vi "Fit EPR Spectra (QSM)-Rev2.vi"(8 "Spectral Data In":T6={"PDT Amp [v]"=0.0, "RIS Amp [v]"=0.0, "B-Field"=[], "All In-Phase Scan Spectra"=[], "Model Select"=enum."OneCompRISTwoPDT", "Fit Each Scan"=FALSE, "PDT Center [g]"=0.0, "In-Phase Average Spectra"=[], "In-Phase Median Spectra"=[], "Out-Phase Median Spectra"=[], "Out-Phase Average Spectra"=[], "Fit Spectra"=[], "Fit No-Baseline Spectra"=[], "All Out-Phase Scan Spectra"=[], "Baseline Offset Correction"=FALSE, "In-Phase Offset [v]"=0.0, "Out-Phase Offset [v]"=0.0, "Ch2 Input\n(Balance)"=[], "Ch3 Input\n(Phase)"=[], "Ch4 Input\n(AFC)"=[], "Fit Pars"=[], "Fit Pars Errors"=[], "Fit Pars Labels"=[], "Raw Scan DAQ Data"=[], "Bad Scans Indicies"=[], "Good In-Phase Scan Spectra"=[], "Good Out-Phase Scan Spectra"=[], "Bad In-Phase Scan Spectra"=[], "Bad Out-Phase Scan Spectra"=[], "Number of bad scans"=0, "Fit History"=[], "PDT Amp. History/Set [v]"=[], "RIS Amp. History/Set [v]"=[], "RIS Amp. History/Scan [v]"=[], "All Shifted B-Fields"=[], "Good Shifted B-Fields"=[], "Ch5 Input\n(SpO2)"=[], "Ch6 Input\n(BPM)"=[], "Global SNR"=0.0, "Fit Error History"=[], "SNR History"=[]} {"Global SNR" min=0.0; "PDT Center [g]" min=0.0; "RIS Amp [v]" min=0.0}, 9 "Measurement Information":T1={"Comments"="", "Directory Input"="", "Data file path"=path "C:/Data/EPR Data", "Scripting File"=path "C:/Data/Configuration Script.csv", "Save Data"=FALSE, "Tooth size (d11) [mm]"=0.0, "Tooth size (d12) [mm]"=0.0, "Tooth size (d21) [mm]"=0.0, "Tooth size (d22) [mm]"=0.0, "Dose of Tooth [Gy]"=0.0, "Safe Shutdown?"=FALSE, "Gases Available"=[], "Database Username"="", "Database Password"="", "Database Login URL"="", "Database Upload URL"="", "Database Success URL"="", "Database XML URL"="", "Database Resonator URL"="", "Session Number"=0, "Set #"=0, "Resonator Operator"="", "Session Type"="", "Tooth/Sample ID"="", "Volunteer ID"="", "Computer Operator"="", "Volunteer Type"="", "Site/Tooth Selection (T8,T9)"="", "Resonator"="", "Measurement Site"="", "Non-standard session?"=FALSE, "EPR DAQ Version"="", "Session Path"=path "C:/Data/EPR Data", "Chosen Applied State"="", "Chosen Initial State"="", "Time of Transition"="", "DAQ Mode"=enum."Engineering", "pO2/Scan [mmHg]"=[], "pO2/Set [mmHg]"=[], "Linewidth (HWHM)/Scan [Gauss]"=[], "Linewidth (HWHM)/Set [Gauss]"=[], "pO2 Conversion"="", "Dose Calibration Cluster"={"Dose Response"={"grand_mean"=0.0292016, "slope"=0.0188720543}, "Dose Correction"={"Sex"=1, "a0"=7.719669421, "a1"=-2.746550736, "a2"=-0.186490355, "a3"=0.041922063, "a4"=-0.849147359, "a5"=0.14330063, "a6"=0.019930219, "A_n"=40.0, "H_n"=10.12, "Dose Correction"=FALSE}, "Dose Reporting"={"Reporting is"=TRUE, "sd_threshold [AU]"=0.06, "sd_model [Gy]"=0.66, "dosimetric_threshold [Gy]"=2.0, "Add intrasession errors is"=FALSE, "Prior Radiation?"=FALSE}}, "OxyChip Slope"=0.0, "OxyChip Intercept"=0.0, "QA Mode"=enum."Select QA Mode", "QA Session?"=FALSE, "Sample Type"=enum."Empty Resonator", "Report pO2/Scan"=FALSE, "Skip End Session Save"=FALSE, "Number of sites"=enum."# Probes", "Recipient Name"="", "Sender Name"="", "Recipient Email"="", "Transition State History"=[], "pO2 Report Times"=[], "Temperature [C]"=0.0, "+Error pO2/Scan [mmHg]"=[], "-Error pO2/Scan [mmHg]"=[], "+Error pO2/Set [mmHg]"=[], "-Error pO2/Set [mmHg]"=[], "Oxy Phase Exclusion Tolerance [rad]"=0.0, "Oxy Center Exclusion Tolerance [%]"=0.0, "Oxy Exclude Unacceptable"=FALSE, "Oxy Unacceptable Estimate Flags"=[], "Save Session PPT"=FALSE, "Flagged Bad Sets"=[]} {"Oxy Center Exclusion Tolerance [%]" format="%#_9g"; "Oxy Phase Exclusion Tolerance [rad]" format="%#_9g"; "Temperature [C]" format="%#_9g"; "OxyChip Intercept" format="%#_9g"; "OxyChip Slope" format="%#_9g"; "Dose Calibration Cluster"."Dose Reporting"."dosimetric_threshold [Gy]" format="%#_9g"; "Dose Calibration Cluster"."Dose Reporting"."sd_model [Gy]" format="%#_9g"; "Dose Calibration Cluster"."Dose Reporting"."sd_threshold [AU]" format="%#_9g"; "Dose Calibration Cluster"."Dose Correction"."H_n" format="%#_9g"; "Dose Calibration Cluster"."Dose Correction"."A_n" format="%#_9g"; "Dose Calibration Cluster"."Dose Correction"."a6" format="%#.9g"; "Dose Calibration Cluster"."Dose Correction"."a5" format="%#.9g"; "Dose Calibration Cluster"."Dose Correction"."a4" format="%#.9g"; "Dose Calibration Cluster"."Dose Correction"."a3" format="%#.9g"; "Dose Calibration Cluster"."Dose Correction"."a2" format="%#.9g"; "Dose Calibration Cluster"."Dose Correction"."a1" format="%#.9g"; "Dose Calibration Cluster"."Dose Correction"."a0" format="%#.9g"; "Dose Calibration Cluster"."Dose Correction"."Sex" items=["Male"=1, "Female"=0]; "Dose Calibration Cluster"."Dose Response"."slope" format="%#_9g"; "Dose Calibration Cluster"."Dose Response"."grand_mean" format="%#_9g"}, 10 "Hardware Parameters In":T5={"Scan Calibration [G/V]"=0.0, "Modulation Calibration [G/V]"=0.0, "Modulation Phase [deg]"=0.0, "Modulation Frequency [Hz]"=0.0, "Attenuation [dB]"=0, "Input Channel Count"=0, "Time constant"=7, "Sensitivity"=17, "Frequency Output Voltage [V]"=0.0, "Phase Output Voltage [V]"=0.0, "Lock-in Offset Compensation"=FALSE, "RF [GHz]"=0.0, "Q Start"=0.0, "Q End"=0.0, "Balance"=0.0, "Phase Error"=0.0, "AFC Error"=0.0, "AFC"=FALSE, "Magnet Rotation"=FALSE, "Balance Scaling Factor"=1.0, "Phase Error Scaling Factor"=1.0, "AFC Error Scaling Factor"=1.0, "Frequency Counter ID"="", "Sweep Waveform"=enum."Sawtooth", "Q-Factor Scale"=0.0, " Q-Data Scale"=0.0, " Q-Data Offset"=0.0, "Magnet Rotation Slope"=0.0, "Magnet Rotation Offset"=0.0, "Phase Sweep Resolution"=0.0, "Hardware Version Number"="", "Spectrometer ID Number"=0, "Spectrometer Name"="", "Lock in Saturation"=0.0, "Balance Threshold"=0.0, "Phase Error Threshold"=0.0, "AFC Error Threshold"=0.0, "Linear Actuator Length"=0.0, "Lock-in OK?"=FALSE, "Ignore Lock-in Comm. Failure"=FALSE, "Gradient Addresses"=[], "Gradient Calibrations [G/A*mm]"=[], "Gradient Power Supplies"=[], "Lock-in Address"="", "Magnet Type"=enum."RRI", "Camera Names"=[], "Sweep Limit [Gauss]"=0.0, "Modulation Limit [Gauss]"=0.0, "Balance Threshold Exceeded?"=FALSE, "Phase Threshold Exceeded?"=FALSE, "AFC Threshold Exceeded?"=FALSE, "Consecutive Re-tune attempts"=0, "Reverse Sweep Slope [sec]"=0.0, "Reverse Sweep Offset [G]"=0.0, "AFC Field Correction [V/MHz]"=0.0, "Active Gradients (X Y Z)"=[], "SpO2 Calibration [SpO2/V]"=1.0, "Heart Rate Calibration [BPM/V]"=1.0, "Thermocouple Channel"=""} {"Sensitivity" items=["10 us", "20 us", "40 us", "80 us", "160 us", "320 us", "640 us", "5 ms", "10 ms", "20 ms", "50 ms", "100 ms", "200 ms", "500 ms", "1 s", "2 s", "5 s", "10 s", "20 s", "50 s", "100 s", "200 s", "500 s", "1 ks", "2 ks", "5 ks", "10 ks", "20 ks", "50 ks", "100 ks"]; "Time constant" items=["10 us", "20 us", "40 us", "80 us", "160 us", "320 us", "640 us", "5 ms", "10 ms", "20 ms", "50 ms", "100 ms", "200 ms", "500 ms", "1 s", "2 s", "5 s", "10 s", "20 s", "50 s", "100 s", "200 s", "500 s", "1 ks", "2 ks", "5 ks", "10 ks", "20 ks", "50 ks", "100 ks"]}, 11 "Acquisition Parameters In":T4={"Magnet Angle [deg]"=0.0, "Magnet Angles [deg]"=[], "DeltaVpp [v]"=0.0, "SEM [v]"=0.0, "DeltaVpp Thresh [v]"=0.0, "SEM Thresh [v]"=2.0, "Adaptive Processing"=FALSE, "Acquire Q"=FALSE, "Acquire Photos"=FALSE, "Adaptive Tuning"=FALSE, "Automated Matching"=FALSE, "X-Gradient [G/mm]"=0.0, "Y-Gradient [G/mm]"=0.0, "Z-Gradient [G/mm]"=0.0, "Central Field [G]"=0.0, "Scan Width [G]"=0.0, "Mod. Amp. [G]"=0.0, "Scan Time [s]"=0.0, "Pre-Scan Delay [ms]"=0, "Measurement Timeout [s]"=0.0, "Electromagnet Main Field [G]"=0.0, "Locked Central Field [G]"=0.0, "Scans Excluded"=0, "Scans Completed"=0, "No. Scans/Set"=0, "No. Scans for SNR"=0, "Field Locked Frequency [GHz]"=0.0, "Auto Set-based Field Center"=FALSE, "Prompt for oxy acquisition updates"=FALSE, "Oxy QA Scan?"=FALSE, "Exclude Bad Data"=FALSE, "Optimizing RF Power"=FALSE, "Gradients on/off"=FALSE, "Running Script"=TRUE, "Opto-Coupler Current [A]"=0.0, "Continuous Sweeping"=FALSE, "Sweep Rise Time [sec]"=0, "Reverse Sweep Central Field [G]"=0.0, "Forward Sweep Central Field [G]"=0.0, "Sweep Calibrated"=FALSE, "Modulation Calibrated"=FALSE, "First CheckCal Scan?"=FALSE, "AFC Field Correction"=FALSE, "OxyQAInit Scan Width [G]"=0.0, "OxyQAInit Mod. Amp. [G]"=0.0, "Scans Completed/Session"=0, "Acquire SpO2"=FALSE, "Acquire Temperature"=FALSE, "Over Mod"=FALSE} {"OxyQAInit Mod. Amp. [G]" min=0.0; "OxyQAInit Scan Width [G]" min=0.0; "Mod. Amp. [G]" min=0.0; "Scan Width [G]" min=0.0; "Central Field [G]" min=0.0; "Measurement Timeout [s]" min=0.0; "Scan Time [s]" min=0.0; "Z-Gradient [G/mm]" min=0.0; "SEM [v]" min=0.0; "DeltaVpp [v]" min=0.0}) -> (0 "Fit Pars and Labels":cluster{"Pars Labels":string[], "pars":dbl[]}, 1 "Spectral Data Out":T6={"PDT Amp [v]"=0.0, "RIS Amp [v]"=0.0, "B-Field"=[], "All In-Phase Scan Spectra"=[], "Model Select"=enum."OneCompRISTwoPDT", "Fit Each Scan"=FALSE, "PDT Center [g]"=0.0, "In-Phase Average Spectra"=[], "In-Phase Median Spectra"=[], "Out-Phase Median Spectra"=[], "Out-Phase Average Spectra"=[], "Fit Spectra"=[], "Fit No-Baseline Spectra"=[], "All Out-Phase Scan Spectra"=[], "Baseline Offset Correction"=FALSE, "In-Phase Offset [v]"=0.0, "Out-Phase Offset [v]"=0.0, "Ch2 Input\n(Balance)"=[], "Ch3 Input\n(Phase)"=[], "Ch4 Input\n(AFC)"=[], "Fit Pars"=[], "Fit Pars Errors"=[], "Fit Pars Labels"=[], "Raw Scan DAQ Data"=[], "Bad Scans Indicies"=[], "Good In-Phase Scan Spectra"=[], "Good Out-Phase Scan Spectra"=[], "Bad In-Phase Scan Spectra"=[], "Bad Out-Phase Scan Spectra"=[], "Number of bad scans"=0, "Fit History"=[], "PDT Amp. History/Set [v]"=[], "RIS Amp. History/Set [v]"=[], "RIS Amp. History/Scan [v]"=[], "All Shifted B-Fields"=[], "Good Shifted B-Fields"=[], "Ch5 Input\n(SpO2)"=[], "Ch6 Input\n(BPM)"=[], "Global SNR"=0.0, "Fit Error History"=[], "SNR History"=[]} {"Global SNR" min=0.0; "PDT Center [g]" min=0.0; "RIS Amp [v]" min=0.0}, 3 "Number of Fit Iterations":i32, 4 "error out":errorcluster, 6 "Global SNR":dbl)   [LabVIEW 2016]
uses:
  Types/Spectral Data.ctl
  Types/Fitting Model Selection.ctl
  Types/Hardware Parameters.ctl
  Types/Acquisition Parameters.ctl
  Types/Measurement Information.ctl
  Dose Calculation and Reporting/Dose Calculation Control.ctl
  Types/Sample Type.ctl
panel:
  # "Session Information"
  # "Oximetric Data and Information"
  # "Email"
  # "Tooth Information"
  # "Database"
  # "Gradients"
  # "Field"
  # "Scans and Sets"
  # "Timing"
  # "Adaptive Dosimetric \nData Processing"
  # "Bridge I/O"
  # "Magnet Rotation"
  # "Field Calibration"
  # "Lock In Amplifier"
  # "Spectrometer Information"
  # "DAQ Settings"
  # "Gradient Coils and Field"
  # "X"
  # "Y"
  # "Z"
  # "Q-Measurements"
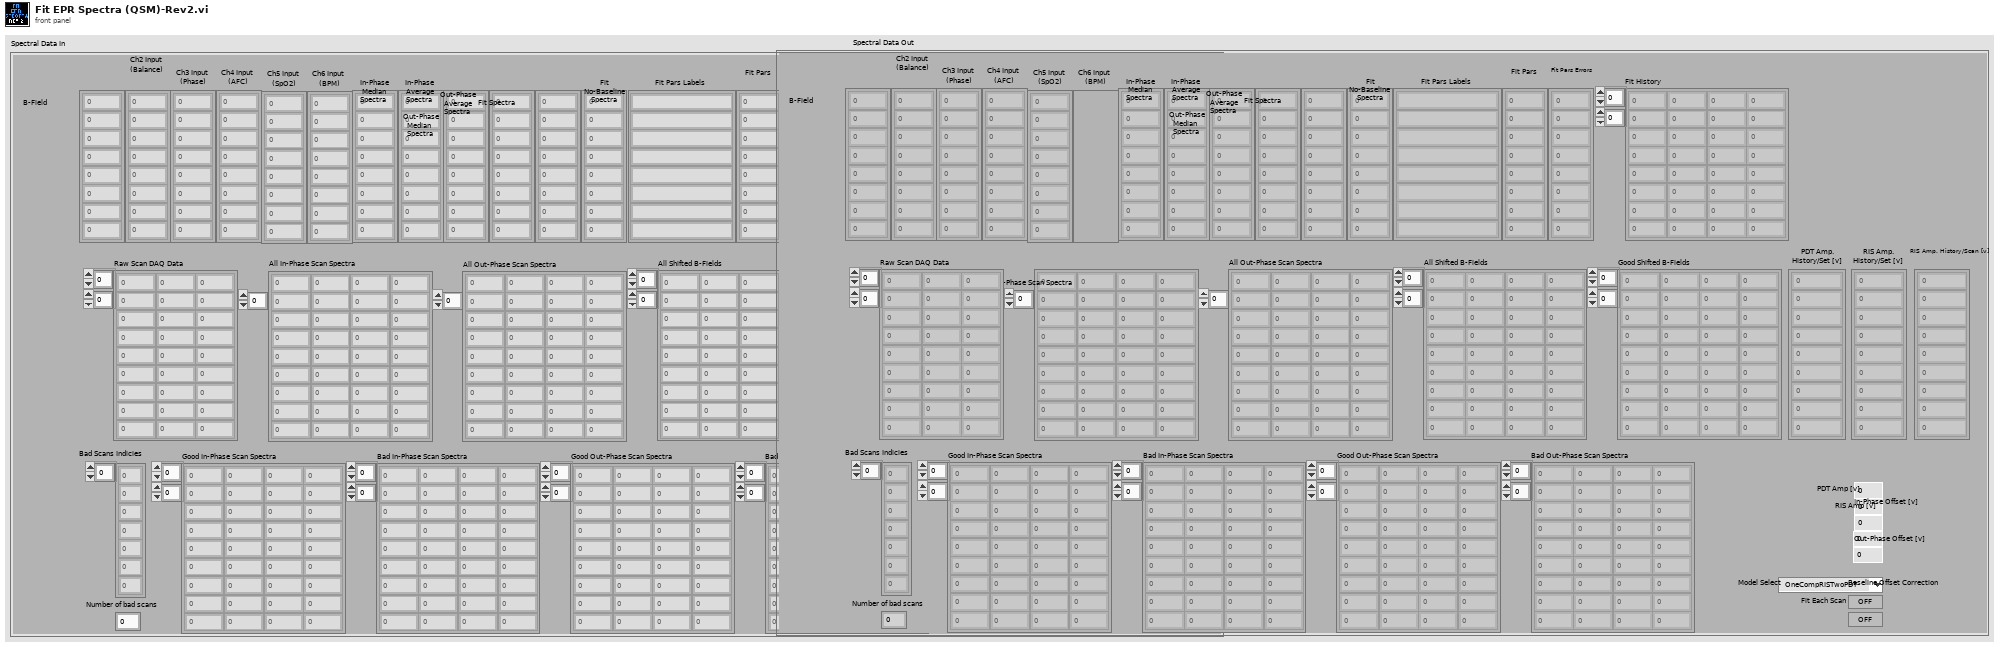
[diagram p1: front panel]
types:
  T1 = typedef "Measurement Information.ctl" = cluster{"Comments":string, "Directory Input":string, "Data file path":path, "Scripting File":path, "Save Data":bool, "Tooth size (d11) [mm]":dbl, "Tooth size (d12) [mm]":dbl, "Tooth size (d21) [mm]":dbl, "Tooth size (d22) [mm]":dbl, "Dose of Tooth [Gy]":dbl, "Safe Shutdown?":bool, "Gases Available":string[], "Database Username":string, "Database Password":string, "Database Login URL":string, "Database Upload URL":string, "Database Success URL":string, "Database XML URL":string, "Database Resonator URL":string, "Session Number":i32, "Set #":u32, "Resonator Operator":string, "Session Type":string, "Tooth/Sample ID":string, "Volunteer ID":string, "Computer Operator":string, "Volunteer Type":string, "Site/Tooth Selection (T8,T9)":string, "Resonator":string, "Measurement Site":string, "Non-standard session?":bool, "EPR DAQ Version":string, "Session Path":path, "Chosen Applied State":string, "Chosen Initial State":string, "Time of Transition":string, "DAQ Mode":enum16{"Engineering", "Dosimetry", "Oximetry"}, "pO2/Scan [mmHg]":dbl[][], "pO2/Set [mmHg]":dbl[][], "Linewidth (HWHM)/Scan [Gauss]":dbl[][], "Linewidth (HWHM)/Set [Gauss]":dbl[][], "pO2 Conversion":string, "Dose Calibration Cluster":T2, "OxyChip Slope":dbl, "OxyChip Intercept":dbl, "QA Mode":enum16{"Select QA Mode", "QA-Start/End", "QA-Mid", "QA-Weekly", "QA-Eng", "Check Calibration"}, "QA Session?":bool, "Sample Type":T3, "Report pO2/Scan":bool, "Skip End Session Save":bool, "Number of sites":enum16{"# Probes", "1", "2", "3", "4"}, "Recipient Name":string, "Sender Name":string, "Recipient Email":string, "Transition State History":string[], "pO2 Report Times":string[], "Temperature [C]":dbl, "+Error pO2/Scan [mmHg]":dbl[][], "-Error pO2/Scan [mmHg]":dbl[][], "+Error pO2/Set [mmHg]":dbl[][], "-Error pO2/Set [mmHg]":dbl[][], "Oxy Phase Exclusion Tolerance [rad]":dbl, "Oxy Center Exclusion Tolerance [%]":dbl, "Oxy Exclude Unacceptable":bool, "Oxy Unacceptable Estimate Flags":bool[], "Save Session PPT":bool, "Flagged Bad Sets":u32[]}
  T2 = typedef "Dose Calculation Control.ctl" = cluster{"Dose Response":cluster{"grand_mean":dbl, "slope":dbl}, "Dose Correction":cluster{"Sex":u16, "a0":dbl, "a1":dbl, "a2":dbl, "a3":dbl, "a4":dbl, "a5":dbl, "a6":dbl, "A_n":dbl, "H_n":dbl, "Dose Correction":bool}, "Dose Reporting":cluster{"Reporting is":bool, "sd_threshold [AU]":dbl, "sd_model [Gy]":dbl, "dosimetric_threshold [Gy]":dbl, "Add intrasession errors is":bool, "Prior Radiation?":bool}}
  T3 = typedef "Sample Type.ctl" = enum16{"Empty Resonator", "IRS", "BallZero", "Irradiated Tooth", "Non-irradiated Tooth", "OxyChip", "LiPc", "PDT", "India Ink"}
  T4 = typedef "Acquisition Parameters.ctl" = cluster{"Magnet Angle [deg]":dbl, "Magnet Angles [deg]":dbl[], "DeltaVpp [v]":dbl, "SEM [v]":dbl, "DeltaVpp Thresh [v]":dbl, "SEM Thresh [v]":dbl, "Adaptive Processing":bool, "Acquire Q":bool, "Acquire Photos":bool, "Adaptive Tuning":bool, "Automated Matching":bool, "X-Gradient [G/mm]":dbl, "Y-Gradient [G/mm]":dbl, "Z-Gradient [G/mm]":dbl, "Central Field [G]":dbl, "Scan Width [G]":dbl, "Mod. Amp. [G]":dbl, "Scan Time [s]":dbl, "Pre-Scan Delay [ms]":u32, "Measurement Timeout [s]":dbl, "Electromagnet Main Field [G]":dbl, "Locked Central Field [G]":dbl, "Scans Excluded":u32, "Scans Completed":u32, "No. Scans/Set":u32, "No. Scans for SNR":u32, "Field Locked Frequency [GHz]":dbl, "Auto Set-based Field Center":bool, "Prompt for oxy acquisition updates":bool, "Oxy QA Scan?":bool, "Exclude Bad Data":bool, "Optimizing RF Power":bool, "Gradients on/off":bool, "Running Script":bool, "Opto-Coupler Current [A]":dbl, "Continuous Sweeping":bool, "Sweep Rise Time [sec]":u32, "Reverse Sweep Central Field [G]":dbl, "Forward Sweep Central Field [G]":dbl, "Sweep Calibrated":bool, "Modulation Calibrated":bool, "First CheckCal Scan?":bool, "AFC Field Correction":bool, "OxyQAInit Scan Width [G]":dbl, "OxyQAInit Mod. Amp. [G]":dbl, "Scans Completed/Session":u32, "Acquire SpO2":bool, "Acquire Temperature":bool, "Over Mod":bool}
  T5 = typedef "Hardware Parameters.ctl" = cluster{"Scan Calibration [G/V]":dbl, "Modulation Calibration [G/V]":dbl, "Modulation Phase [deg]":dbl, "Modulation Frequency [Hz]":dbl, "Attenuation [dB]":u16, "Input Channel Count":i32, "Time constant":u16, "Sensitivity":u16, "Frequency Output Voltage [V]":dbl, "Phase Output Voltage [V]":dbl, "Lock-in Offset Compensation":bool, "RF [GHz]":dbl, "Q Start":dbl, "Q End":dbl, "Balance":dbl, "Phase Error":dbl, "AFC Error":dbl, "AFC":bool, "Magnet Rotation":bool, "Balance Scaling Factor":dbl, "Phase Error Scaling Factor":dbl, "AFC Error Scaling Factor":dbl, "Frequency Counter ID":string, "Sweep Waveform":enum16{"Sine Wave", "Square Wave", "Sawtooth", "Triangle Wave"}, "Q-Factor Scale":dbl, " Q-Data Scale":dbl, " Q-Data Offset":dbl, "Magnet Rotation Slope":dbl, "Magnet Rotation Offset":dbl, "Phase Sweep Resolution":dbl, "Hardware Version Number":string, "Spectrometer ID Number":i32, "Spectrometer Name":string, "Lock in Saturation":dbl, "Balance Threshold":dbl, "Phase Error Threshold":dbl, "AFC Error Threshold":dbl, "Linear Actuator Length":dbl, "Lock-in OK?":bool, "Ignore Lock-in Comm. Failure":bool, "Gradient Addresses":string[], "Gradient Calibrations [G/A*mm]":dbl[], "Gradient Power Supplies":string[], "Lock-in Address":refnum<visa-resource-name>, "Magnet Type":enum16{"RRI", "BARDA", "Whole Body Permanent", "RRI Electromagnet"}, "Camera Names":string[], "Sweep Limit [Gauss]":dbl, "Modulation Limit [Gauss]":dbl, "Balance Threshold Exceeded?":bool, "Phase Threshold Exceeded?":bool, "AFC Threshold Exceeded?":bool, "Consecutive Re-tune attempts":i32, "Reverse Sweep Slope [sec]":dbl, "Reverse Sweep Offset [G]":dbl, "AFC Field Correction [V/MHz]":dbl, "Active Gradients (X Y Z)":bool[], "SpO2 Calibration [SpO2/V]":dbl, "Heart Rate Calibration [BPM/V]":dbl, "Thermocouple Channel":tag}
  T6 = typedef "Spectral Data.ctl" = cluster{"PDT Amp [v]":dbl, "RIS Amp [v]":dbl, "B-Field":dbl[], "All In-Phase Scan Spectra":dbl[][], "Model Select":T7, "Fit Each Scan":bool, "PDT Center [g]":dbl, "In-Phase Average Spectra":dbl[], "In-Phase Median Spectra":dbl[], "Out-Phase Median Spectra":dbl[], "Out-Phase Average Spectra":dbl[], "Fit Spectra":dbl[], "Fit No-Baseline Spectra":dbl[], "All Out-Phase Scan Spectra":dbl[][], "Baseline Offset Correction":bool, "In-Phase Offset [v]":dbl, "Out-Phase Offset [v]":dbl, "Ch2 Input\n(Balance)":dbl[], "Ch3 Input\n(Phase)":dbl[], "Ch4 Input\n(AFC)":dbl[], "Fit Pars":dbl[], "Fit Pars Errors":dbl[], "Fit Pars Labels":string[], "Raw Scan DAQ Data":dbl[][], "Bad Scans Indicies":i32[], "Good In-Phase Scan Spectra":dbl[][], "Good Out-Phase Scan Spectra":dbl[][], "Bad In-Phase Scan Spectra":dbl[][], "Bad Out-Phase Scan Spectra":dbl[][], "Number of bad scans":i32, "Fit History":dbl[][], "PDT Amp. History/Set [v]":dbl[], "RIS Amp. History/Set [v]":dbl[], "RIS Amp. History/Scan [v]":dbl[], "All Shifted B-Fields":dbl[][], "Good Shifted B-Fields":dbl[][], "Ch5 Input\n(SpO2)":dbl[], "Ch6 Input\n(BPM)":dbl[], "Global SNR":dbl, "Fit Error History":dbl[][], "SNR History":dbl[]}
  T7 = typedef "Fitting Model Selection.ctl" = enum16{"OneCompRIS", "OneCompRISTwoPDT", "OneCompRISRev", "OneCompRISTwoPDTRev", "LiPc", "TwoLiPc", "ThreeLiPc", "FourLiPc", "PDTCalibration", "CE_Ink", "Printex", "MelaninTwoPDT"}
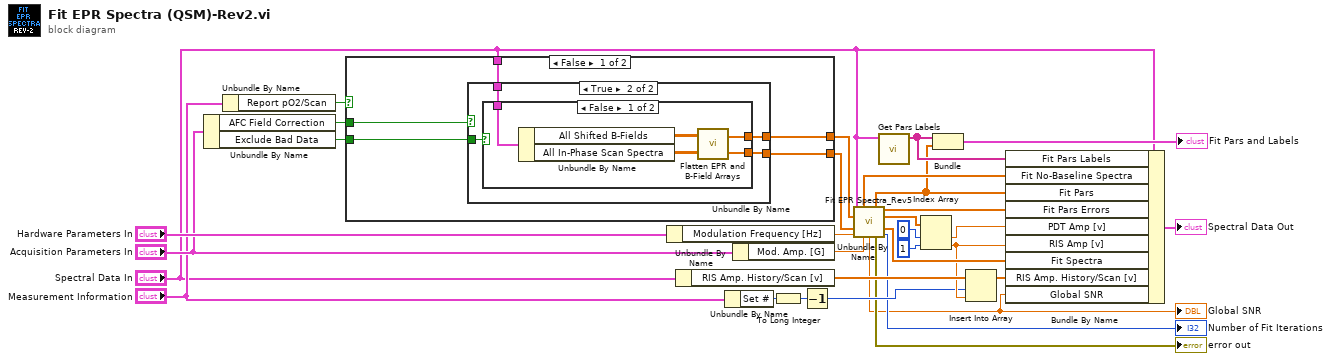
[diagram p0: block diagram]
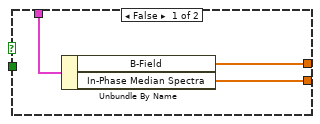
[diagram p2: hidden frame]
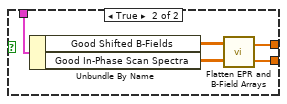
[diagram p3: hidden frame]
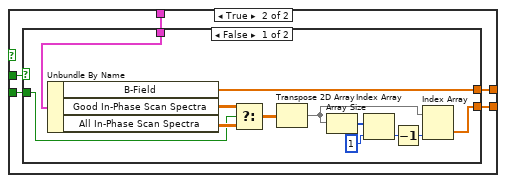
[diagram p4: hidden frame]
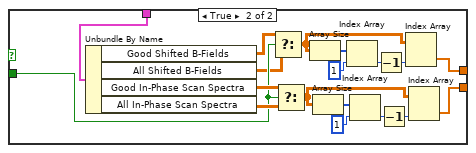
[diagram p5: hidden frame]
diagram:
  n1 = Unbundle By Name("Acquisition Parameters In") -> ("AFC Field Correction"=w10:bool, "Exclude Bad Data"=w9:bool)
  n2 = Unbundle By Name("Measurement Information") -> ("Report pO2/Scan"=w8:bool)
  n3 = case shown="False" w8 {
    tunnel: w10 -> [w36 w56]
    tunnel: w9 -> [w35 w55]
    tunnel: [w34 w58] -> w6
    tunnel: [w33 w57] -> w5
    tunnel: "Spectral Data In" -> [w32 w54]
    frame False {
      n4 = case shown="True" w36 {
        tunnel: w35 -> [_ w43]
        tunnel: [w39 w42] -> w34
        tunnel: [w38 w41] -> w33
        tunnel: w32 -> [w37 w40]
        frame False {
          n5 = Unbundle By Name(w37) -> ("B-Field"=w39:dbl[], "In-Phase Median Spectra"=w38:dbl[])
        }
        frame True {
          n6 = case shown="False" w43 {
            tunnel: [w47 w52] -> w42
            tunnel: [w45 w50] -> w41
            tunnel: w40 -> [w44 w49]
            frame False {
              n7 = Unbundle By Name(w44) -> ("All Shifted B-Fields"=w48:dbl[][], "All In-Phase Scan Spectra"=w46:dbl[][])
              n8 = call "Flatten EPR and B-Field Arrays.vi"("2D EPR Data"=w46, "2D B-Fields"=w48) -> ("1D Flattened EPR Data"=w45:dbl[], "1D Flattened B-Fields"=w47:dbl[])
            }
            frame True {
              n9 = Unbundle By Name(w49) -> ("Good Shifted B-Fields"=w53:dbl[][], "Good In-Phase Scan Spectra"=w51:dbl[][])
              n10 = call "Flatten EPR and B-Field Arrays.vi"("2D EPR Data"=w51, "2D B-Fields"=w53) -> ("1D Flattened EPR Data"=w50:dbl[], "1D Flattened B-Fields"=w52:dbl[])
            }
          }
        }
      }
    }
    frame True {
      n11 = case shown="False" w56 {
        tunnel: w55 -> [w61 w75]
        tunnel: [w70 w76] -> w58
        tunnel: [w65 w84] -> w57
        tunnel: w54 -> [w60 w71]
        frame False {
          n12 = Unbundle By Name(w60) -> ("B-Field"=w70:dbl[], "Good In-Phase Scan Spectra"=w64:dbl[][], "All In-Phase Scan Spectra"=w62:dbl[][])
          n13 = Select(t=w64, s=w61, f=w62) -> (s? t:f=w63:dbl[][])
          n14 = Transpose 2D Array(2D array=w63) -> (transposed array=w59:dbl[][])
          n15 = Array Size(array=w59) -> (size(s)=w66:i32[])
          n16 = Index Array(array=w66, index=1) -> (element=w68:i32)
          n17 = Decrement(x=w68) -> (x-1=w69:i32)
          n18 = Index Array(array=w59, index (col)=w69) -> (element=w65:dbl[])  [unwired: 1 in]
        }
        frame True {
          n19 = Unbundle By Name(w71) -> ("Good Shifted B-Fields"=w74:dbl[][], "All Shifted B-Fields"=w73:dbl[][], "Good In-Phase Scan Spectra"=w83:dbl[][], "All In-Phase Scan Spectra"=w81:dbl[][])
          n20 = Select(t=w74, s=w75, f=w73) -> (s? t:f=w72:dbl[][])
          n21 = Select(t=w83, s=w75, f=w81) -> (s? t:f=w82:dbl[][])
          n22 = Array Size(array=w72) -> (size(s)=w80:i32[])
          n23 = Array Size(array=w82) -> (size(s)=w85:i32[])
          n24 = Index Array(array=w80, index=1) -> (element=w78:i32)
          n25 = Index Array(array=w85, index=1) -> (element=w87:i32)
          n26 = Decrement(x=w78) -> (x-1=w77:i32)
          n27 = Decrement(x=w87) -> (x-1=w88:i32)
          n28 = Index Array(array=w72, index (col)=w77) -> (element=w76:dbl[])  [unwired: 1 in]
          n29 = Index Array(array=w82, index (col)=w88) -> (element=w84:dbl[])  [unwired: 1 in]
        }
      }
    }
  }
  n30 = Unbundle By Name("Hardware Parameters In") -> ("Modulation Frequency [Hz]"=w30:dbl)
  n31 = Unbundle By Name("Spectral Data In") -> ("RIS Amp. History/Scan [v]"=w16:dbl[])
  n32 = Unbundle By Name("Measurement Information") -> ("Set #"=w15:u32)
  n33 = Unbundle By Name("Acquisition Parameters In") -> ("Mod. Amp. [G]"=w29:dbl)
  n34 = To Long Integer(number=w15) -> (32bit integer=w14:i32)
  n35 = Decrement(x=w14) -> (x-1=w7:i32)
  n36 = call "Fit EPR Spectra_Rev5.vi"("Spectral Data In"="Spectral Data In", "B"=w6, "y"=w5, "modFreq"=w30, "modAmp"=w29) -> ("fitNoBaseline"=w27:dbl[], "pars"=w19:dbl[], "parsError"=w26:dbl[], "vpp"=w25:dbl[], "fit"=w21:dbl[], "Global SNR"=w1:dbl, "error out"=→"error out":errorcluster, "Number of Fit Iterations"=→"Number of Fit Iterations":i32)  [unwired: 3 in]
  "Global SNR" <- w1
  n37 = call "Get Pars Labels.vi"("Spectral Data In"="Spectral Data In") -> ("Pars Labels"=w20:string[])  [unwired: 10 in]
  n38 = Index Array(array=w25, index #1=0 ("index"), index #2=1 ("index")) -> (element #1=w22:dbl, element #2=w13:dbl)
  n39 = Bundle("Pars Labels"=w20, "pars"=w19) -> (→"Fit Pars and Labels":cluster{"Pars Labels":string[], "pars":dbl[]})  [unwired: 1 in]
  n40 = Insert Into Array(array=w16, index=w7, new element=w13) -> (w17:dbl[])
  n41 = Bundle By Name(cluster="Spectral Data In", "Fit Pars Labels"=w20, "Fit No-Baseline Spectra"=w27, "Fit Pars"=w19, "Fit Pars Errors"=w26, "PDT Amp [v]"=w22, "RIS Amp [v]"=w13, "Fit Spectra"=w21, "RIS Amp. History/Scan [v]"=w17, "Global SNR"=w1) -> (→"Spectral Data Out":T6)
